vi "motor XY setMeng.vi"(6 "Motor settings Z":cluster{"Vmax (mm/s)":sgl, "Acc (mm/s/s)":sgl}, 8 "Enum in":enum16{"Int", "Set"}(ring), 9 "Motor settings (X,Y)":cluster{"Vmax (mm/s)":sgl, "Acc (mm/s/s)":sgl}, 10 "Array":errorcluster[](array[cluster]), 11 "Array 2":refnum<k7>[](array[refnum])) -> (0 "Enum out":enum16{"Int", "Set"}(ring), 1 "Array 3":errorcluster[](array[cluster]), 3 "Array 4":refnum<k7>[](array[refnum]))   [LabVIEW 2014]
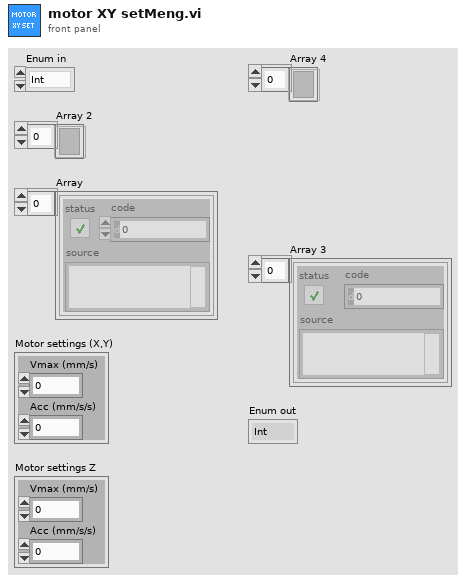
[diagram p1: front panel]
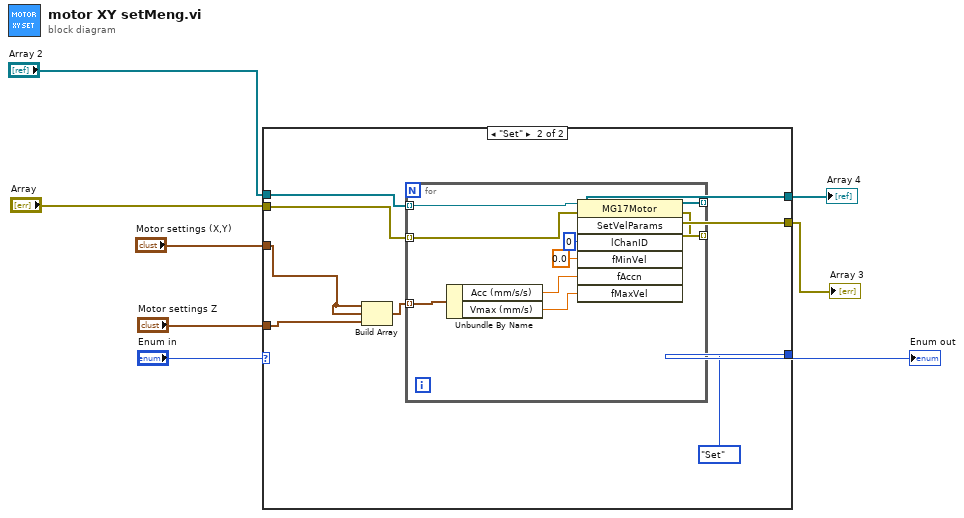
[diagram p0: block diagram]
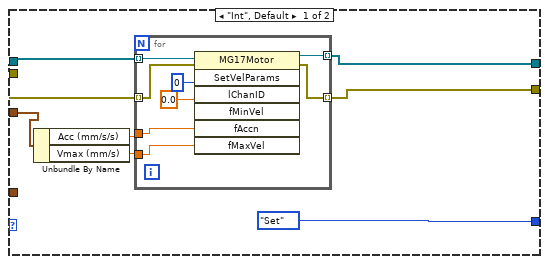
[diagram p2: hidden frame]
diagram:
  n1 = case shown="\"Set\"" "Enum in" {
    tunnel: [w11 w28] -> w3
    tunnel: [w10 w31] -> w1
    tunnel: "Array" -> [w16 w32]
    tunnel: [enum16{"Int", "Set"}."Set" ("Enum") enum16{"Int", "Set"}."Set" ("Enum")] -> w6
    tunnel: "Array 2" -> [w12 w29]
    tunnel: "Motor settings (X,Y)" -> [w9 w27]
    tunnel: "Motor settings Z" -> [_ w26]
    frame "Int", Default {
      n2 = Unbundle By Name(w9) -> ("Acc (mm/s/s)"=w15:sgl, "Vmax (mm/s)"=w14:sgl)
      n3 = for {
        tunnel: w15 -> [w18]
        tunnel: w14 -> [w17]
        tunnel: w12 -> [w24] mode=indexing
        tunnel: [w21] -> w11 mode=indexing
        tunnel: w16 -> [w20] mode=indexing
        tunnel: [w19] -> w10 mode=indexing
        n4 = invoke class="MG17Motor" method="SetVelParams"(reference=w24, error in=w20, "lChanID"=0, "fMinVel"=sgl 0.0, "fAccn"=w18, "fMaxVel"=w17) -> (reference out=w21:refnum<k7>, error out=w19:errorcluster)  [unwired: 1 in, 5 out]
      }
    }
    frame "Set" {
      n5 = Build Array(w27, w27, w26) -> (w25:cluster{"Vmax (mm/s)":sgl, "Acc (mm/s/s)":sgl}[])
      n6 = for {
        tunnel: w29 -> [w40] mode=indexing
        tunnel: w32 -> [w41] mode=indexing
        tunnel: [w37] -> w28 mode=indexing
        tunnel: [w36] -> w31 mode=indexing
        tunnel: w25 -> [w35] mode=indexing
        n7 = Unbundle By Name(w35) -> ("Acc (mm/s/s)"=w34:sgl, "Vmax (mm/s)"=w33:sgl)
        n8 = invoke class="MG17Motor" method="SetVelParams"(reference=w40, error in=w41, "lChanID"=0, "fMinVel"=sgl 0.0, "fAccn"=w34, "fMaxVel"=w33) -> (reference out=w37:refnum<k7>, error out=w36:errorcluster)  [unwired: 1 in, 5 out]
      }
    }
  }
  "Array 3" <- w1
  "Array 4" <- w3
  "Enum out" <- w6
